vi "niScope EX Getting Started.vi"() -> ()   [LabVIEW 2021]
doc: "Example: Getting Started\n\nRecommended Input Signal: 100 kHz, 1.8 Vpp, sine wave\n\nDevices Supported: Refer to NI Example Finder\n\nLabVIEW Description:\n\nThis example opens a session to the NI-SCOPE driver by passing in the device's resource name to the Initialize VI. The resource name is a unique identifier for your National Instruments' hardware product. It can be found (and changed) by running Measurement & Automation Explorer (MAX). A shortcut to MAX is placed on your desktop when NI-SCOPE or NI-DAQ is installed.\n\nThe session handle returned from the Initialize VI is a parameter to all VIs in the NI-SCOPE driver. Only one session may be opened at a time for your oscilloscope, and every session should be closed by calling the Close vi. The session should be closed even when an error occurs.\n\nThe Auto Setup VI takes several acquisitions to measure the amplitude and frequency of the input signal. This allows it to optimally set properties such as the sample rate, vertical range, and minimum record length. The Read VI, initiates an acquisition, waits for it to finish, and fetches the data from the oscilloscope. The data is returned as a bundle of the initial x, x increment, and waveform. Initial x is the time of the first point in the waveform relative to the trigger, while the x increment is the time between two points in the waveform. This bundle may be directly wired to a waveform graph, to display the waveform with timing information. \n\nThe Error Handler VI translates any error messages into text messages."
uses:
  <instrlib>/niScope/Acquire/niScope Multi Read Cluster.vi
  <instrlib>/niDigital/niDigital.llb/niDigital Selected Function.ctl
  <instrlib>/niDigital/niDigital.llb/niDigital Get Site Results Site Numbers.vi
  <instrlib>/niDigital/niDigital.llb/niDigital Burst Pattern (Pass Fail).vi
panel:
  in  "error in":errorcluster
  out "error out":errorcluster
  out "Site":string[](array[string])
  out "Pass?":bool[](array[boolean])
  in  "Digital":refnum<k15>="PXI1Slot2,PXI1Slot3" caption="resource name"
  out "Waveform Graph":T1(graph)
  in  "Scope":refnum<k15>="Dev1" caption="Resource Name(s)"
  in  "Scope Channel(s)":string="0"
  # "Overview: Demonstrates the minimal code needed to use NI-SCOPE.\nRequirements: NI-SCOPE\nInstructions: \n1.  Select the appropriate device in the Resource Name control.\n2.  Enter the channels you would like to acquire from in the Channel(s) control.\n3.  Run the VI."
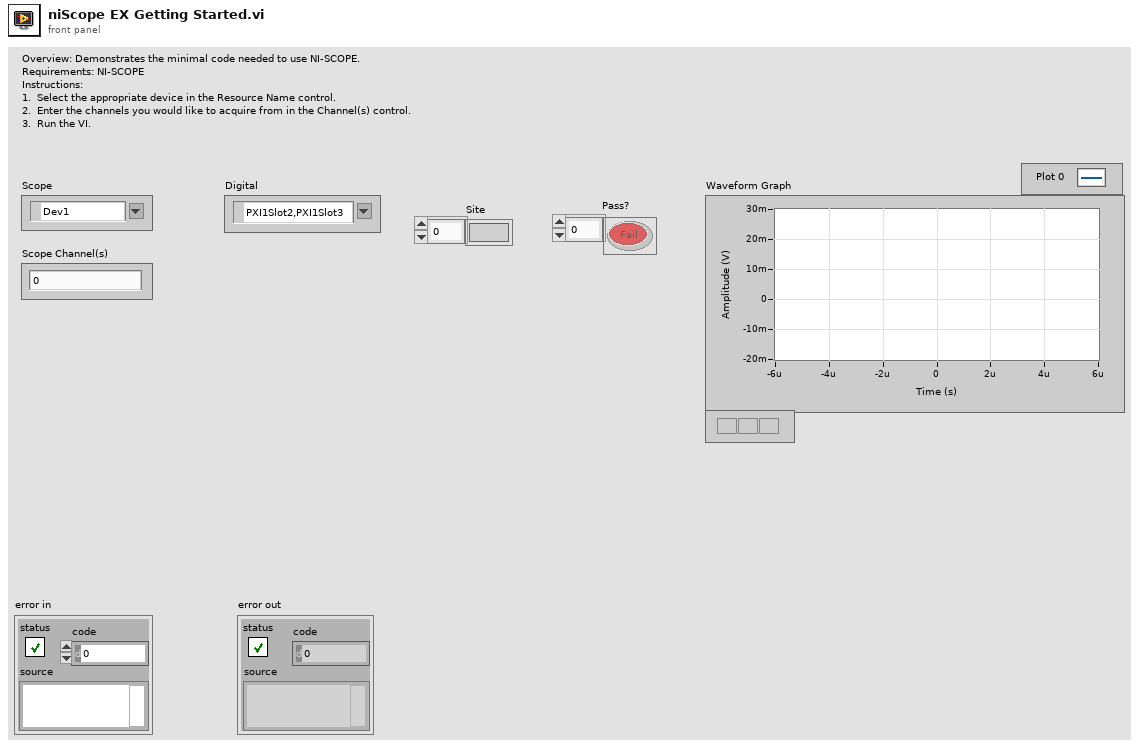
[diagram p1: front panel]
types:
  T1 = cluster{"relativeInitialX":dbl, "xIncrement":dbl, "wfm":dbl[]}[]
  T2 = typedef "niDigital Selected Function.ctl" = i32
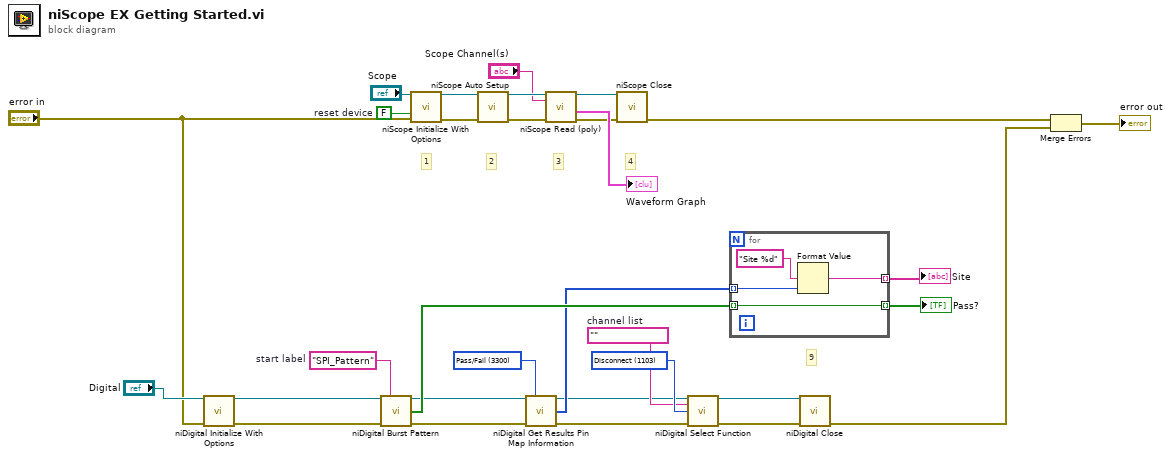
[diagram p0: block diagram]
diagram:
  w14 = ""  # channel list
  w15 = T2 1103 items=["Digital"=1100, "PPMU"=1101, "Off"=1102, "Disconnect"=1103] ("function")
  w20 = "SPI_Pattern"  # start label
  w16 = 3300 items=["Pass/Fail"=3300, "Capture Waveform"=3301] ("site result type")
  w28 = FALSE  # reset device
  # "9"
  # "4"
  # "3"
  # "2"
  # "1"
  n1 = call <instrlib>:"niDigital Initialize With Options.vi"("resource name"="Digital", "error in"="error in") -> ("instrument handle"=w8:refnum<k15>, "error out"=w7:errorcluster)  [unwired: 12 in]
  n2 = call-poly <instrlib>:"niDigital Burst Pattern.vi"("instrument handle"=w8, "start label"=w20, "error in"=w7) -> ("instrument handle out"=w19:refnum<k15>, "pass"=w21:bool[], "error out"=w18:errorcluster)  [unwired: 10 in]
  n3 = call <instrlib>:"niScope Initialize With Options.vi"("resource name"="Scope", "reset device"=w28, "error in"="error in") -> ("instrument handle"=w31:refnum<k15>, "error out"=w30:errorcluster)  [unwired: 11 in]
  n4 = call <instrlib>:"niScope Auto Setup.vi"("instrument handle"=w31, "error in"=w30) -> ("instrument handle out"=w27:refnum<k15>, "error out"=w26:errorcluster)  [unwired: 12 in]
  n5 = call-poly <instrlib>:"niDigital Get Results Pin Map Information.vi"("instrument handle"=w19, "site result type"=w16, "error in"=w18) -> ("instrument handle out"=w13:refnum<k15>, "site numbers"=w17:i32[], "error out"=w12:errorcluster)  [unwired: 10 in]
  n6 = call-poly <instrlib>:"niScope Read (poly).vi"("error in"=w26, "channels"="Scope Channel(s)", "instrument handle"=w27) -> ("error out"=w23:errorcluster, "waveform"=→"Waveform Graph":T1, "instrument handle out"=w22:refnum<k15>)  [unwired: 5 in, 1 out]
  n7 = call <instrlib>:"niScope Close.vi"("instrument handle"=w22, "error in"=w23) -> ("error out"=w4:errorcluster)  [unwired: 13 in]
  n8 = call <instrlib>:"niDigital Select Function.vi"("instrument handle"=w13, "channel list"=w14, "function"=w15, "error in"=w12) -> ("instrument handle out"=w10:refnum<k15>, "error out"=w11:errorcluster)  [unwired: 10 in]
  n9 = for {
    tunnel: w21 -> [w32] mode=indexing
    tunnel: w17 -> [w34] mode=indexing
    tunnel: [w33] -> w6 mode=indexing
    tunnel: [w32] -> w5 mode=indexing
    n10 = Format Value(format string="Site %d", value (0)=w34) -> (output string=w33:string)  [unwired: 1 in]
  }
  "Pass?" <- w5
  "Site" <- w6
  n11 = call <instrlib>:"niDigital Close.vi"("instrument handle"=w10, "error in"=w11) -> ("error out"=w2:errorcluster)  [unwired: 13 in]
  n12 = Merge Errors(w4, w2) -> (→"error out":errorcluster)
